vi "Dummy-DoesNothing.vi"() -> (0 "New Values In":string[][](array[string]), 1 "New Chs In":string[](array[string]))   [LabVIEW 2022 SP3]
uses:
  Results_plotter_Global.vi
  Data plotting/subVIs/Plot_Values_Global.vi
panel:
  out "OrdinateStrings":string[](array[string])
  out "legends":string[](array[string])
  out "plottedChannel":string[](array[string])
  out "graphSeries":cluster{"Xvalues":dbl[], "Yvalues":dbl[]}[](array[cluster])
  # "This VI receives does nothing- just illustrates what you can receive from the RFP global and work with.\n\nUse as a starting point to devlop new calculation plugins, or as a convenient way to cancel if you accidentally pressed \"Calculate new metadata\"!"
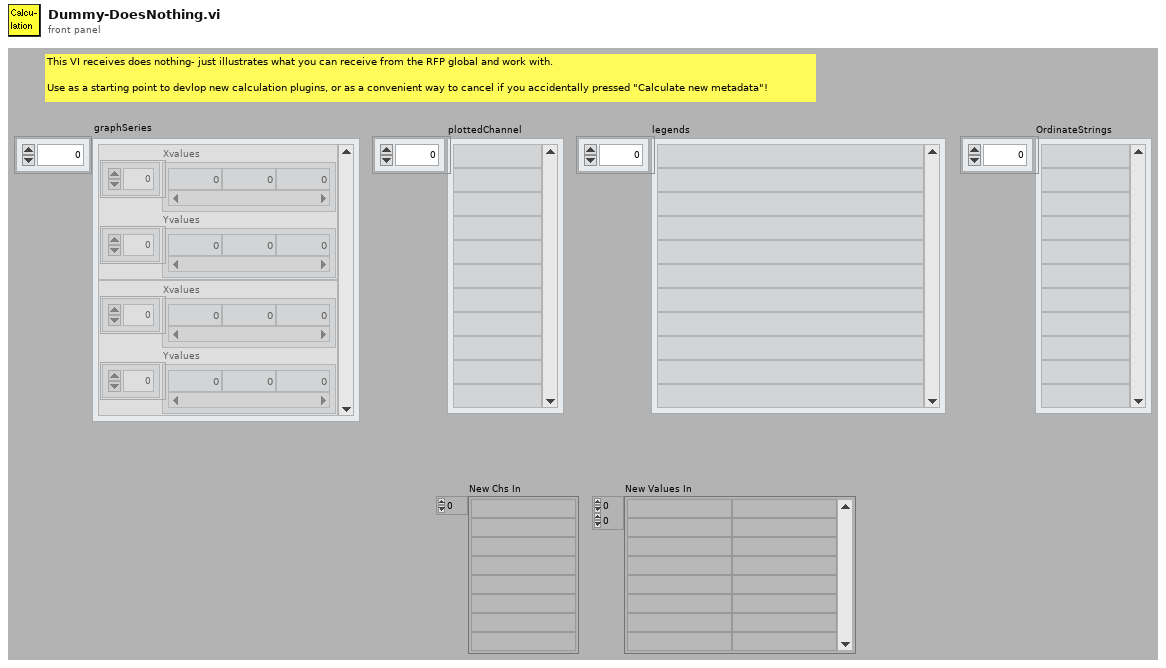
[diagram p1: front panel]
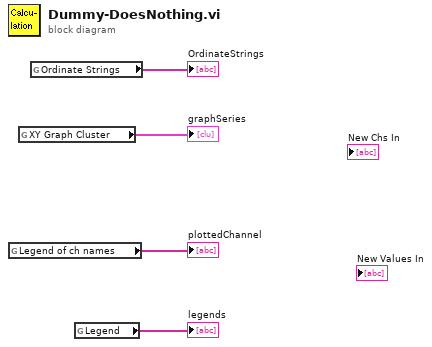
[diagram p0: block diagram]
diagram:
  n1 = global read "Results_plotter_Global.vi" "Legend of ch names"() -> (→"plottedChannel":string[])
  n2 = global read "Plot_Values_Global.vi" "XY Graph Cluster"() -> (→"graphSeries":cluster{dbl[], dbl[]}[])
  n3 = global read "Results_plotter_Global.vi" "Ordinate Strings"() -> (→"OrdinateStrings":string[])
  n4 = global read "Results_plotter_Global.vi" "Legend"() -> (→"legends":string[])
